vi "Nearest_neighbors(CuLab).vi"(8 "error in":errorcluster, 9 "n neighbors":i32, 10 "Membank":T1, 11 "Features":refnum<class "T2D_SGL.lvclass">) -> (0 "error out":errorcluster, 3 "patch scores":refnum<class "T1D_SGL.lvclass">, 5 "dT_Nearest_Neighbourrs":dbl)   [LabVIEW 2020]
uses:
  <vilib>/Ngene/CuLab - GPU Accelerated Toolkit/Toolkit/Low_Level/Tensor_Classes/T_Children/T2D/T2D_Children/T2D_SGL/T2D_SGL.lvclass
  C:/Program Files/National Instruments/LabVIEW 2020/vi.lib/Ngene/CuLab - GPU Accelerated Toolkit/Toolkit/Low_Level/Tensor_Classes/T_Children/T2D/T2D.lvclass
  <vilib>/Ngene/CuLab - GPU Accelerated Toolkit/Toolkit/Low_Level/Tensor_Classes/T_Children/T1D/T1D_Children/T1D_SGL/T1D_SGL.lvclass
  API/Controls/MemBank_and_Norm_Variants.ctl
  <vilib>/Ngene/CuLab - GPU Accelerated Toolkit/Toolkit/API/Array/Array Size/CU_Array_Size_T2D.vi
  <vilib>/Ngene/CuLab - GPU Accelerated Toolkit/Toolkit/API/Array/Reshape Array  (API)/CU_Reshape_to_T1D/T2D/CU_Reshape_to_T1D_(T2D_SGL).vi
  <vilib>/Ngene/CuLab - GPU Accelerated Toolkit/Toolkit/API/Signal Processing/Signal Operation/Decimate (single shot) adaptive/CU_Decimate_Single_Shot_Adaptive_T1D_SGL.vi
  <vilib>/Ngene/CuLab - GPU Accelerated Toolkit/Toolkit/CuLab.lvlib
  <vilib>/Ngene/Deep Learning Toolkit/Toolkit/Deep_Learning_Toolkit_by_Ngene.lvlib
  C:/Program Files/National Instruments/LabVIEW 2020/vi.lib/Ngene/CuLab - GPU Accelerated Toolkit/Toolkit/Low_Level/Tensor_Classes/Tensor.lvclass
  C:/Program Files/National Instruments/LabVIEW 2020/vi.lib/Ngene/CuLab - GPU Accelerated Toolkit/Toolkit/Low_Level/Tensor_Classes/T_Children/T2D/T2D_Children/T2D_SGL/T2D_SGL.lvclass
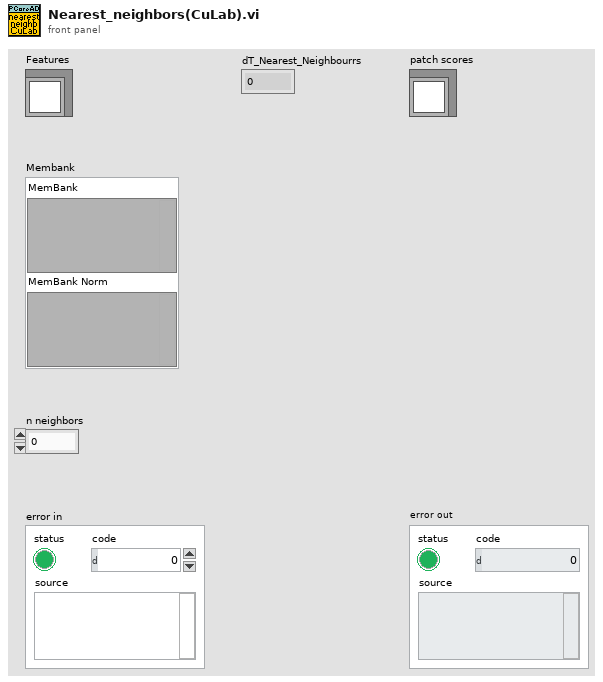
[diagram p1: front panel]
types:
  T1 = typedef "MemBank_and_Norm_Variants.ctl" = cluster{"MemBank":variant, "MemBank Norm":variant}
  T2 = typedef "CuLab.lvlib/T2D_Dims.ctl" = cluster{"H":i32, "W":i32}
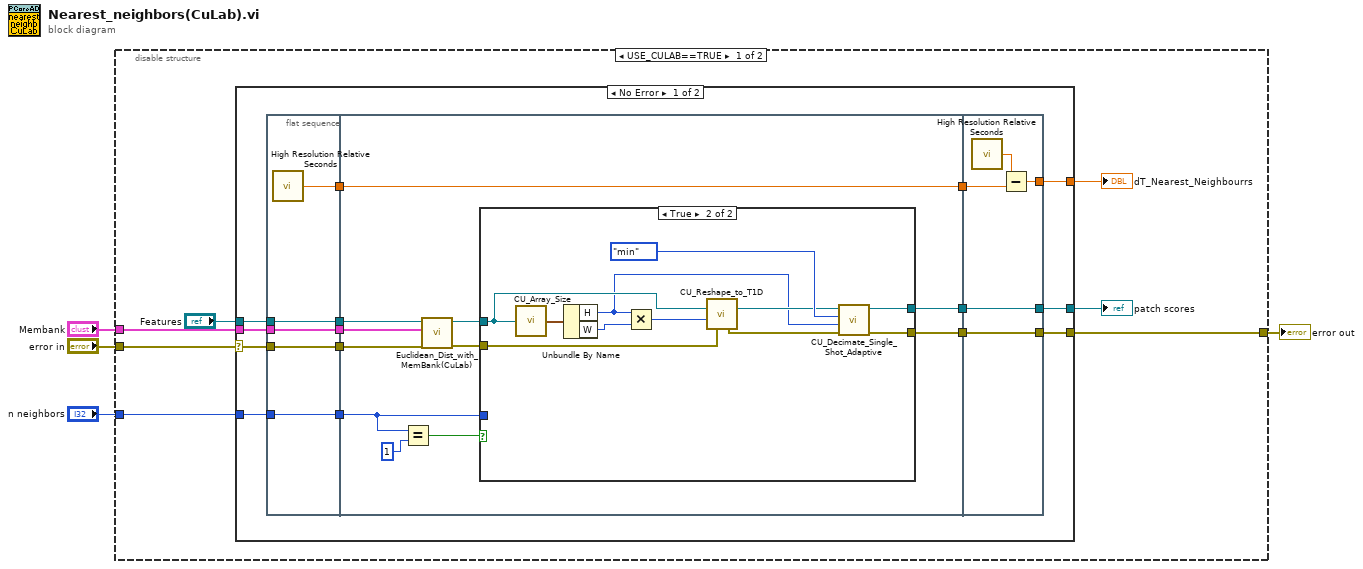
[diagram p0: block diagram]
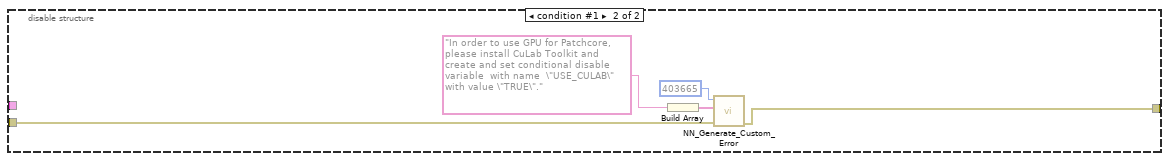
[diagram p4: hidden frame]
diagram:
  n1 = disable-structure shown="USE_CULAB==TRUE" {
    disable-tunnel: "Membank" -> [w8 _]
    disable-tunnel: "error in" -> [w7 w62]
    disable-tunnel: "n neighbors" -> [w6 _]
    disable-tunnel: [w5 w61] -> w1
    frame condition #0 (active) {
      n2 = case shown="No Error" w7 {
        selector: w7 -> [w16 w60]
        tunnel: w6 -> [w19 _]
        tunnel: "Features" -> [w18 _]
        tunnel: w8 -> [w17 _]
        tunnel: [w15 w60] -> w5
        tunnel: [w13 _] -> w10
        tunnel: [w12 _] -> w9
        frame No Error {
          n3 = flat-sequence {
            tunnel: w16 -> [w28]
            tunnel: w17 -> [w29]
            tunnel: w18 -> [w30]
            tunnel: w19 -> [w31]
            tunnel: [w31] -> w26
            tunnel: [w30] -> w25
            tunnel: [w29] -> w24
            tunnel: [w28] -> w23
            tunnel: [w27] -> w22
            tunnel: w26 -> [w42]
            tunnel: w25 -> [w41]
            tunnel: w24 -> [w40]
            tunnel: w23 -> [w37]
            tunnel: w22 -> [w35]
            tunnel: [w35] -> w21
            tunnel: [w34] -> w20
            tunnel: [w33] -> w14
            tunnel: w21 -> [w58]
            tunnel: w20 -> [w57]
            tunnel: [w57] -> w15
            tunnel: w14 -> [w56]
            tunnel: [w56] -> w13
            tunnel: [w55] -> w12
            frame #0 {
              n4 = call <vilib>:"High Resolution Relative Seconds.vi"() -> ("relative seconds"=w27:dbl)
            }
            frame #1 {
              n5 = Equal?(x=w42, y=1) -> (x = y?=w38:bool)
              n6 = call "Euclidean_Dist_with_MemBank(CuLab).vi"("error in"=w37, "Membank"=w40, "x"=w41) -> ("error out"=w36:errorcluster, "Distances"=w32:refnum<class "T2D_SGL.lvclass">)  [unwired: 6 in, 1 out]
              n7 = case shown="True" w38 {
                tunnel: w42 -> [_ _]
                tunnel: w32 -> [_ w54]
                tunnel: w36 -> [w43 w46]
                tunnel: [w43 w45] -> w34
                tunnel: [_ w44] -> w33
                frame False {
                }
                frame True {
                  n8 = call-poly <vilib>:"CU_Array_Size.vi"("Tensor"=w54) -> ("T2D_Dims"=w53:T2)  [unwired: 14 in]
                  n9 = Unbundle By Name(w53) -> ("H"=w48:i32, "W"=w51:i32)
                  n10 = Multiply(x=w48, y=w51) -> (x*y=w50:i32)
                  n11 = call-poly <vilib>:"CU_Reshape_to_T1D.vi"("Tensor in"=w54, "Dest Dim"=w50, "error in (no error)"=w46) -> ("Dest out"=w49:refnum<class "T1D_SGL.lvclass">, "error out"=w47:errorcluster)  [unwired: 11 in]
                  n12 = call-poly <vilib>:"CU_Decimate_Single_Shot_Adaptive.vi"("error in (no error)"=w47, "output size"=w48, "operation"=enum16{"avg", "min", "max", "maxmin"}."min", "X"=w49) -> ("error out"=w45:errorcluster, "Y"=w44:refnum<class "T1D_SGL.lvclass">)  [unwired: 6 in]
                }
              }
            }
            frame #2 {
              n13 = call <vilib>:"High Resolution Relative Seconds.vi"() -> ("relative seconds"=w59:dbl)
              n14 = Subtract(x=w59, y=w58) -> (x-y=w55:dbl)
            }
          }
        }
        frame Error {
        }
      }
      "patch scores" <- w10
      "dT_Nearest_Neighbourrs" <- w9
    }
    frame condition #1 {
      n15 = Build Array("In order to use GPU for Patchcore, please install CuLab Toolkit and create and set conditional disable variable  with name  \"USE_CULAB\" with value \"TRUE\"." ("Message")) -> (w64:string[])
      n16 = call <vilib>:"NN_Generate_Custom_Error.vi"("error in (no error)"=w62, "Message"=w64, "Error_code"=403665) -> ("error out"=w61:errorcluster)  [unwired: 8 in]
    }
  }
  "error out" <- w1
